vi "Resolve Glyph.vi"(7 "Size":dbl=16.0, 8 "error in (no error)":errorcluster, 10 "Glyph Name":string, 11 "LV-Awesome.lvlib:LV Awesome.lvclass":refnum<class "LV Awesome.lvclass">) -> (0 "error out":errorcluster, 1 "charcode":u32 format="%x", 2 "Font Settings out":refnum<class "Font Settings.lvclass">, 3 "LV-Awesome.lvlib:LV Awesome.lvclass 2":refnum<class "LV Awesome.lvclass">)   [LabVIEW 2023, in "LV-Awesome.lvlib" / "LV Awesome.lvclass"]
uses:
  LV Awesome/LV Awesome.lvclass
  Font Glyph Drawer Interface/Font Settings/Font Settings.lvclass
  LV Awesome/LV Awesome.lvclass/LV Awesome.ctl
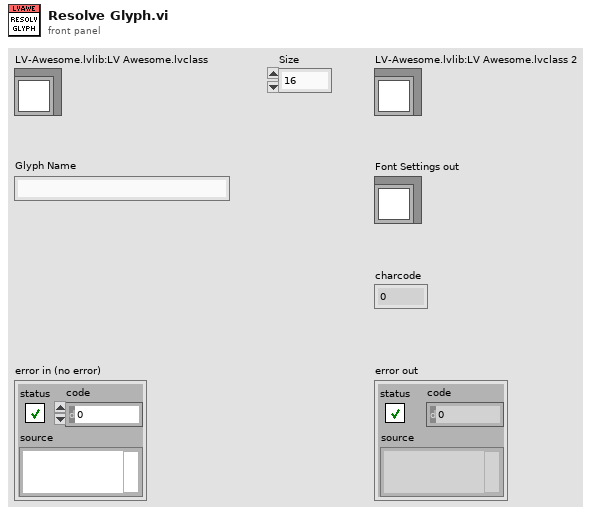
[diagram p1: front panel]
types:
  T1 = typedef "LV-Awesome.lvlib/LV Awesome.lvclass/Data.ctl" = cluster{"Glyphs":map{string, u32}, "Fonts":map{string, path}}
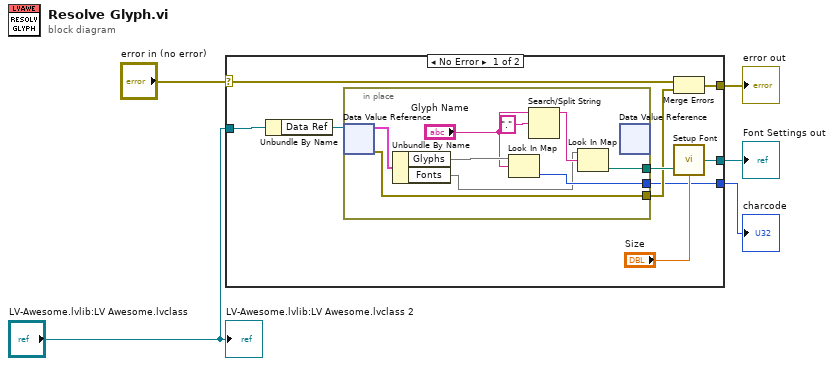
[diagram p0: block diagram]
diagram:
  n1 = case shown="No Error" "error in (no error)" {
    selector: "error in (no error)" -> [w7 w24]
    tunnel: "LV-Awesome.lvlib:LV Awesome.lvclass" -> [w14 _]
    tunnel: [w12 _] -> w4
    tunnel: [w9 w24] -> w3
    tunnel: [w6 _] -> w1
    frame No Error {
      n2 = Unbundle By Name(w14) -> ("Data Ref"=w11:refnum<data-value>)
      n3 = in-place {
        in-place-border: [w21] -> w6
        in-place-border: [w17] -> w10
        in-place-border: [w16] -> w8
        n4 = in-place-dvr #1(w11) -> (w20:T1, w16:errorcluster)
        n5 = Unbundle By Name(w20) -> ("Glyphs"=w19:map{string, u32}, "Fonts"=w18:map{string, path})
        n6 = Look In Map(map=w19, key="Glyph Name") -> (value=w21:u32)  [unwired: 1 in, 1 out]
        n7 = Search/Split String(string="Glyph Name", search string/char (-)=".") -> (substring before match=w23:string)  [unwired: 1 in, 2 out]
        n8 = Look In Map(map=w18, key=w23) -> (value=w17:path)  [unwired: 1 in, 1 out]
        n9 = in-place-dvr #1() -> ()  [unwired: 1 in, 2 out]
      }
      n10 = Merge Errors(w7, w8) -> (w9:errorcluster)
      n11 = call "Setup Font.vi"("Size"="Size", "Font Path (System)"=w10) -> ("Font Settings out"=w12:refnum<class "Font Settings.lvclass">)  [unwired: 1 in]
    }
    frame Error {
    }
  }
  "Font Settings out" <- w4
  "error out" <- w3
  "charcode" <- w1
  "LV-Awesome.lvlib:LV Awesome.lvclass 2" <- "LV-Awesome.lvlib:LV Awesome.lvclass"
